vi "sendMode.vi"(8 "error in (no error)":errorcluster, 9 "Function":i32, 10 "Address":i32, 11 "Mockbus in":refnum<class "Mockbus.lvclass">) -> (0 "error out":errorcluster, 3 "Mockbus out":refnum<class "Mockbus.lvclass">)   [LabVIEW 2015, in "Mockbus.lvclass"]
uses:
  Mockbus.lvclass
  Mockbus.lvclass/Mockbus.ctl
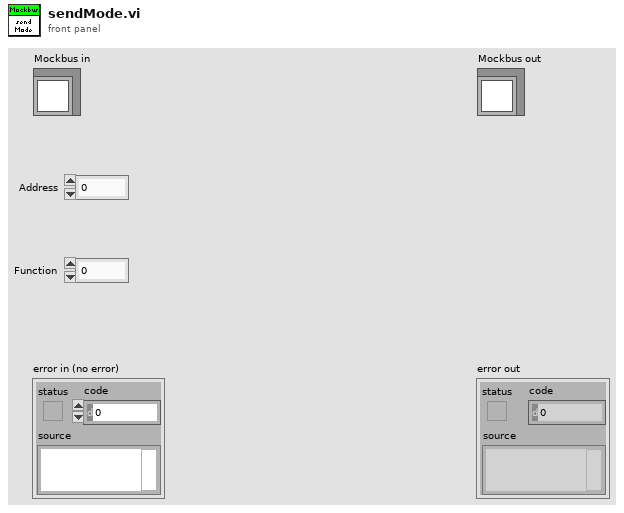
[diagram p1: front panel]
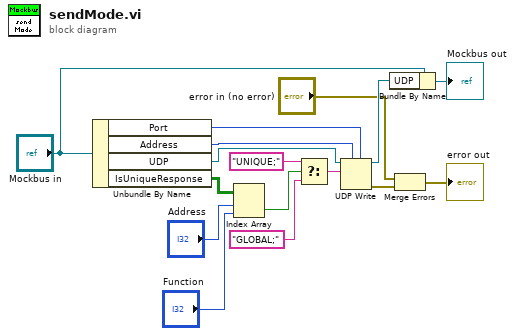
[diagram p0: block diagram]
diagram:
  n1 = Unbundle By Name("Mockbus in") -> ("Port"=w14:u16, "Address"=w15:u32, "UDP"=w16:refnum<k16>, "IsUniqueResponse"=w7:bool[][])
  n2 = Index Array(array=w7, index (row)="Address", index (col)="Function") -> (element=w4:bool)
  n3 = Select(t="UNIQUE;", s=w4, f="GLOBAL;") -> (s? t:f=w1:string)
  n4 = UDP Write(address=w15, port or service name=w14, connection ID=w16, data in=w1) -> (error out=w11:errorcluster, 3:w12:refnum<k16>)  [unwired: 2 in]
  n5 = Bundle By Name(cluster="Mockbus in", "UDP"=w12) -> (→"Mockbus out":refnum<class "Mockbus.lvclass">)
  n6 = Merge Errors("error in (no error)", w11) -> (→"error out":errorcluster)
